vi "Periodic Tasks.vi"(8 "error in":errorcluster) -> ()   [LabVIEW 2015]
doc: "This VI runs in parallel to other tasks. It can contain as many user-defined periodic loops as you need. These can carry out PID or other sorts of timed response."
uses:
  <vilib>/Rock Robotics/WPI/Solenoid/WPI_SolenoidValue.ctl
  <vilib>/Rock Robotics/WPI/Utilities/WPI_GetSetVariantRefNum.vi
  Robot Global Data.vi
  <vilib>/Rock Robotics/WPI/Solenoid/WPI_SolenoidSetEnum.vi
  <vilib>/Rock Robotics/Network Tables/NT Write Number.vi
  <vilib>/Rock Robotics/Network Tables/NT Write Boolean.vi
  <vilib>/Rock Robotics/WPI/Solenoid/Deprecated/WPI_SolenoidGetBool.vi
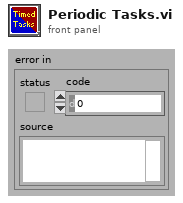
[diagram p1: front panel]
types:
  T1 = typedef "WPI_JoystickDevRef.ctl" = cluster{"Device":T2}
  T2 = typedef "WPI_JoystickDeviceEnum.ctl" = enum16{"USB 0", "USB 1", "USB 2", "USB 3", "USB 4", "USB 5"}
  T3 = typedef "WPI_SolenoidValue.ctl" = enum16{"Off", "On", "Forward", "Reverse"}
  T4 = typedef "WPI_SolenoidDevRef.ctl" = cluster{"DevStatus":errorcluster, "Pneumatics Control Module":u8, "Forward Solenoid Channel":T5, "Reverse Solenoid Channel":T5}
  T5 = typedef "WPI_SolenoidChannel.ctl" = enum8{"Solenoid 0", "Solenoid 1", "Solenoid 2", "Solenoid 3", "Solenoid 4", "Solenoid 5", "Solenoid 6", "Solenoid 7", "Invalid"}
  T6 = typedef "WPI_RobotDriveDevRef.ctl" = cluster{"DevStatus":errorcluster, "Motors[]":T7[], "Square Inputs":bool, "Max Output":dbl}
  T7 = typedef "WPI_MotorControlDeviceRef.ctl" = cluster{"DeviceStatus":errorcluster, "Type":T8, "PWM":cluster{"PWM Channel":T9, "DeadBand":T10}, "CAN":cluster{"Device Number":u8, "Control Mode":T11, "Semaphore":T12, "Max Vout":dbl, "TalonSRX Control Mode":T13}, "Invert":bool}
  T8 = typedef "WPI_MotorControlType.ctl" = enum16{"PWM", "CAN", "CANTalonSRX"}
  T9 = typedef "FPGA_DIOPWMChannel.ctl" = enum8{"PWM 0", "PWM 1", "PWM 2", "PWM 3", "PWM 4", "PWM 5", "PWM 6", "PWM 7", "PWM 8", "PWM 9", "PWM MXP 0", "PWM MXP 1", "PWM MXP 2", "PWM MXP 3", "PWM MXP 4", "PWM MXP 5", "PWM MXP 6", "PWM MXP 7", "PWM MXP 8", "PWM MXP 9", "Invalid"}
  T10 = typedef "WPI_PWMDeadband.ctl" = cluster{"Name":string, "maxPositivePwm":i32, "minPositivePwm":i32, "centerPwm":i32, "maxNegativePwm":i32, "minNegativePwm":i32, "angularRange":u16}
  T11 = typedef "WPI_CANJaguar_ControlMode.ctl" = enum8{"Percent VBus", "Current", "Speed", "Position", "Voltage"}
  T12 = typedef "Semaphore RefNum" = refnum<k1>
  T13 = typedef "WPI_CANTalonSRX_APIControlMode.ctl" = enum8{"Percent VBus", "Speed", "Position", "Slave", "Unchanged / Invalid", "Voltage Compensation", "Current", "Motion Profile"}
  T14 = cluster{"JoystickDevRef":T1, "RobotDriveDevRef":T6}
  T15 = typedef "WPI_CompressorDevRef.ctl" = cluster{"DevStatus":errorcluster, "Pneumatics Control Module":u8}
  T16 = typedef "WPI_DigitalInputDevRef.ctl" = cluster{"DevStatus":errorcluster, "DIO Channel":T17}
  T17 = typedef "FPGA_DIOChannel.ctl" = enum8{"DIO 0", "DIO 1", "DIO 2", "DIO 3", "DIO 4", "DIO 5", "DIO 6", "DIO 7", "DIO 8", "DIO 9", "DIO MXP 0", "DIO MXP 1", "DIO MXP 2", "DIO MXP 3", "DIO MXP 4", "DIO MXP 5", "DIO MXP 6", "DIO MXP 7", "DIO MXP 8", "DIO MXP 9", "DIO MXP 10", "DIO MXP 11", "DIO MXP 12", "DIO MXP 13", "DIO MXP 14", "DIO MXP 15", "Invalid"}
  T18 = typedef "WPI_AnalogChannelDevRef.ctl" = cluster{"DevStatus":errorcluster, "Analog Channel":T19}
  T19 = typedef "FPGA_AIChannel.ctl" = enum8{"AI 0", "AI 1", "AI 2", "AI 3", "AI MXP 0", "AI MXP 1", "AI MXP 2", "AI MXP 3", "Invalid"}
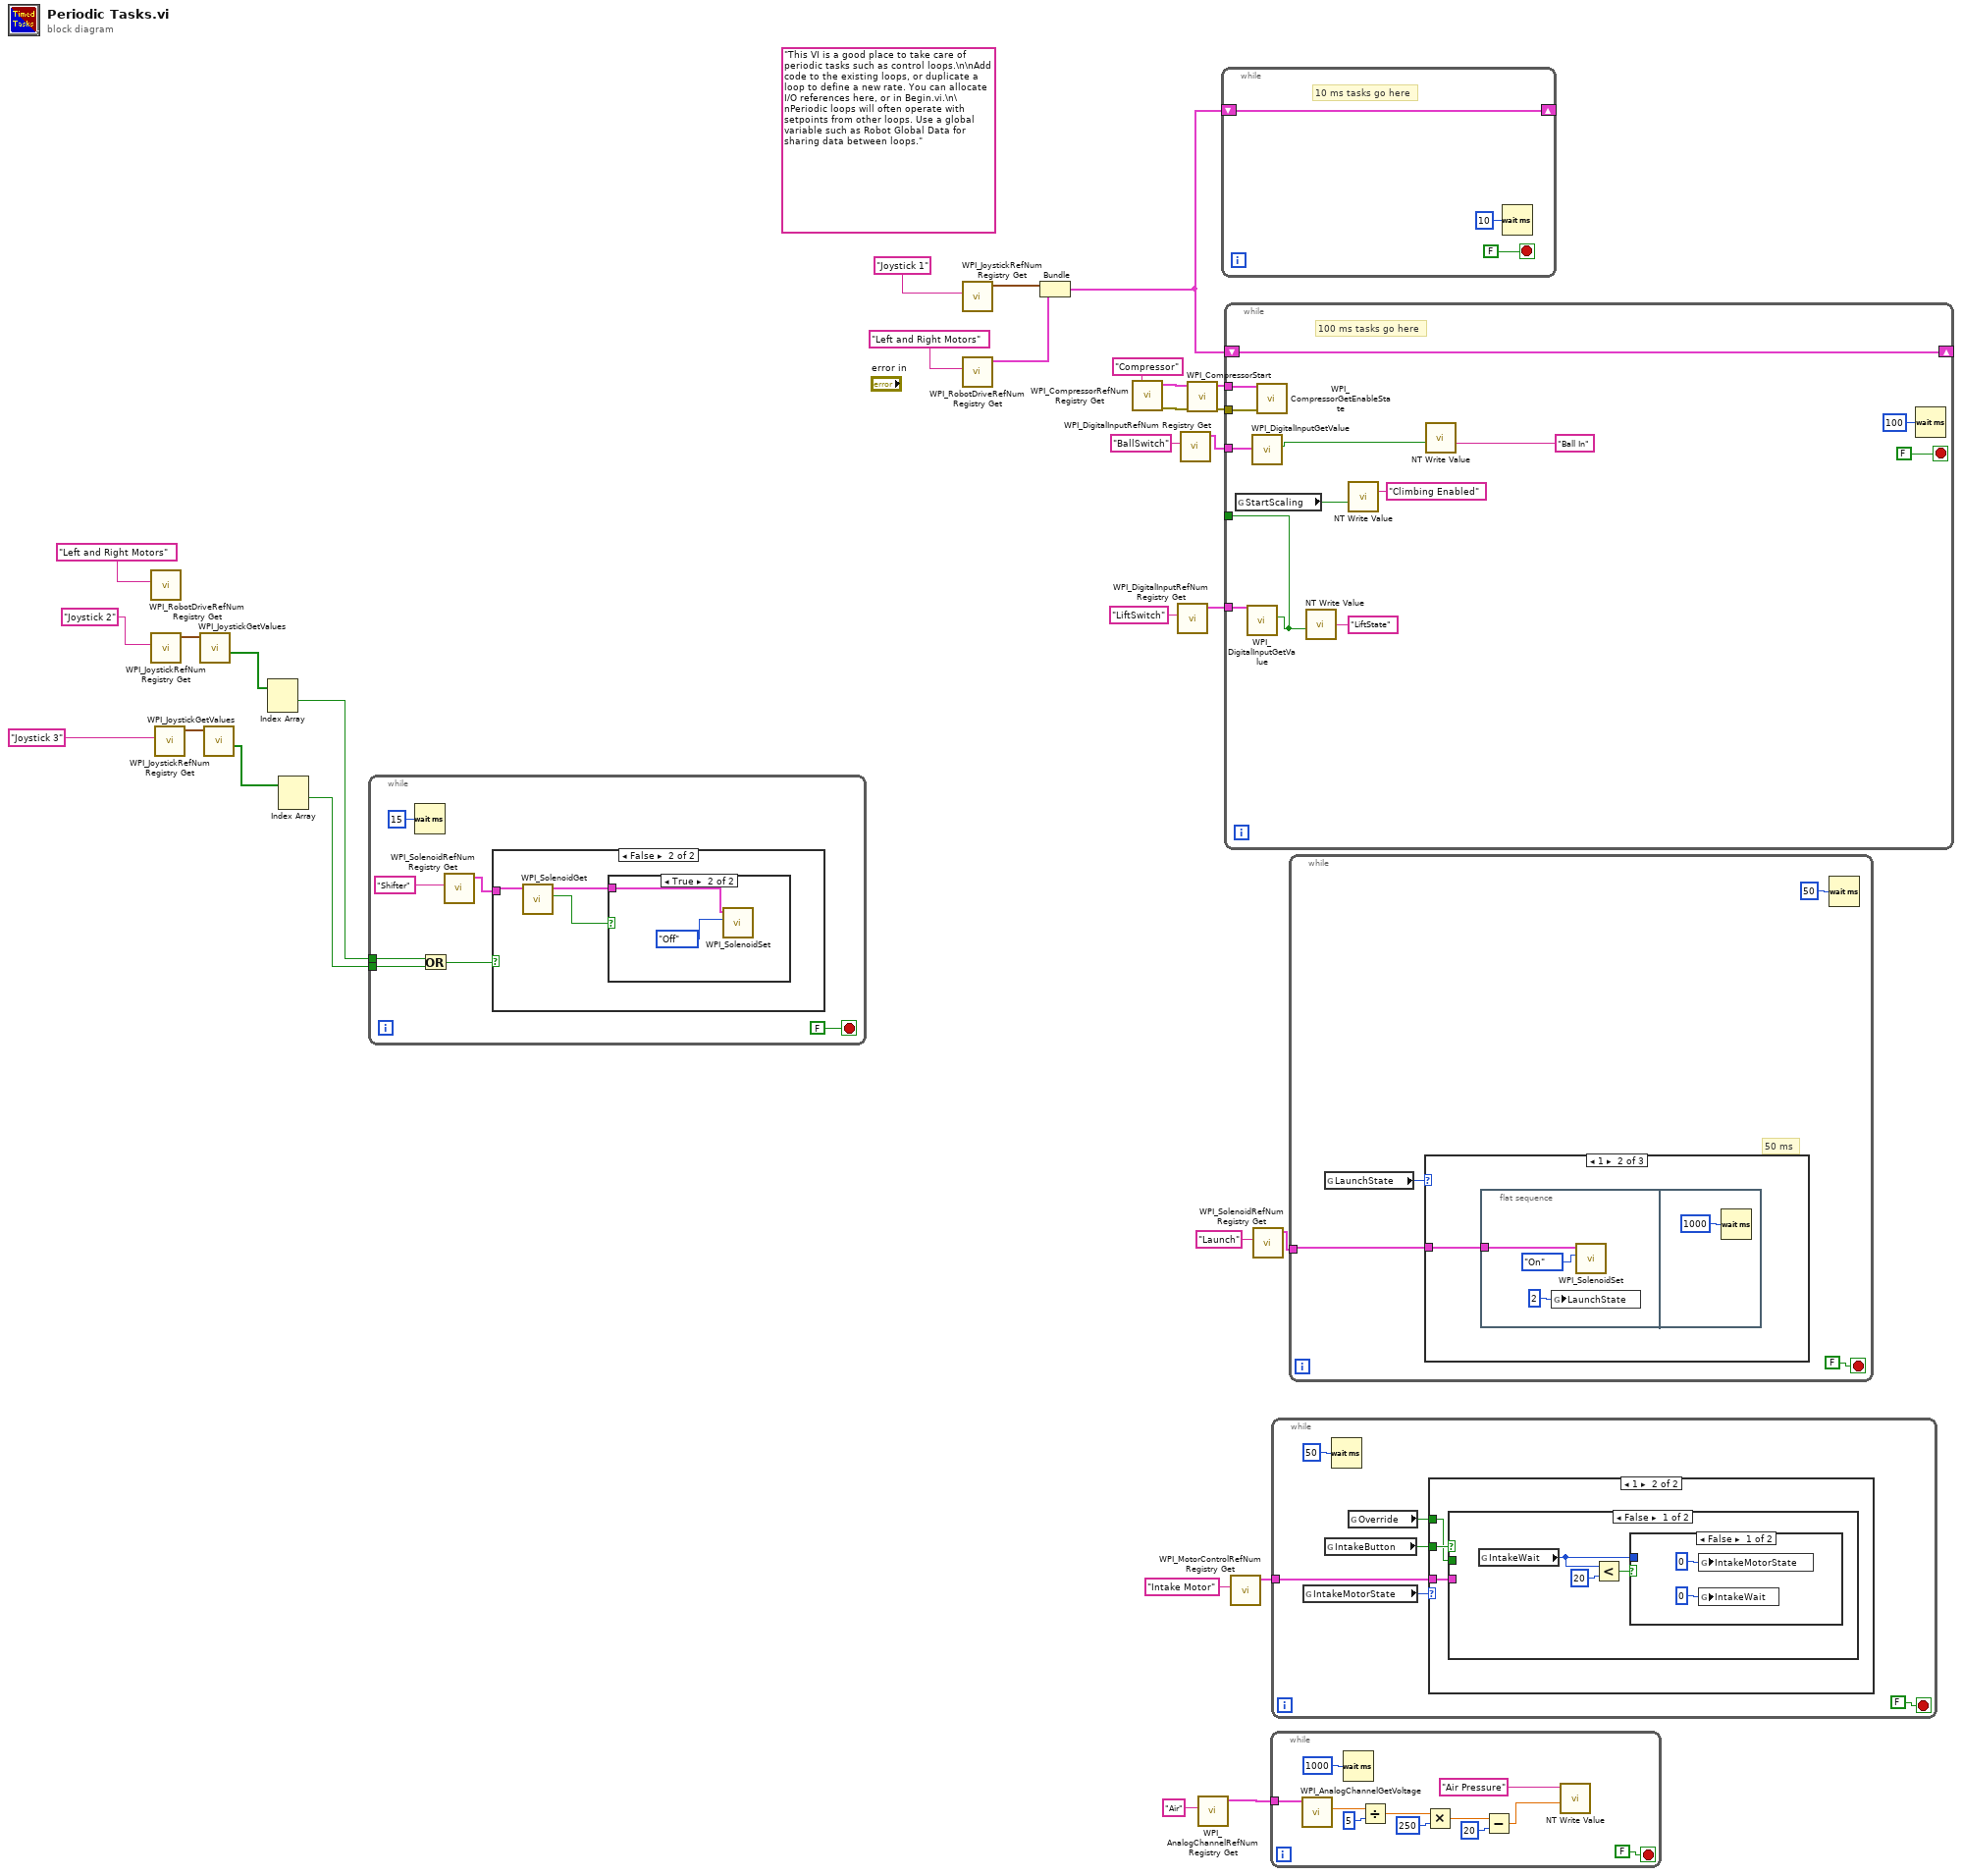
[diagram p0: block diagram]
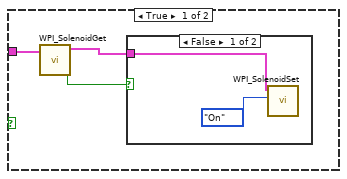
[diagram p2: hidden frame]
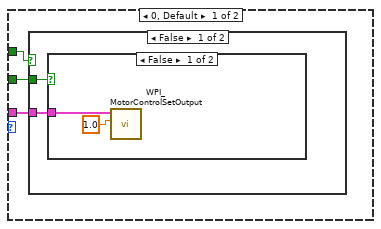
[diagram p5: hidden frame]
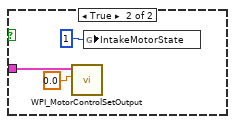
[diagram p6: hidden frame]
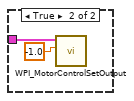
[diagram p7: hidden frame]
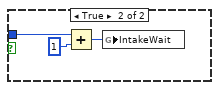
[diagram p8: hidden frame]
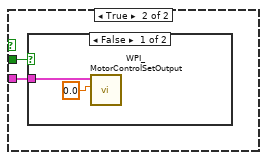
[diagram p9: hidden frame]
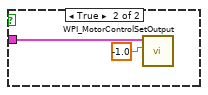
[diagram p10: hidden frame]
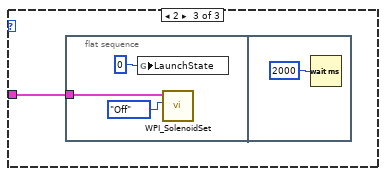
[diagram p12: hidden frame]
diagram:
  (unwired) "This VI is a good place to take care of periodic tasks such as control loops.\n\nAdd code to the existing loops, or duplicate a loop to define a new rate. You can allocate I/O references here, or in Begin.vi.\n\nPeriodic loops will often operate with setpoints from other loops. Use a global variable such as Robot Global Data for sharing data between loops."
  n1 = call <vilib>:"WPI_RobotDriveRefNum Registry Get.vi"("refnum name"="Left and Right Motors") -> ()  [unwired: 1 in, 10 out]
  n2 = call <vilib>:"WPI_JoystickRefNum Registry Get.vi"("refnum name"="Joystick 2") -> ("JoystickDevRef"=w7:T1)  [unwired: 1 in, 9 out]
  n3 = call <vilib>:"WPI_JoystickRefNum Registry Get.vi"("refnum name"="Joystick 3") -> ("JoystickDevRef"=w6:T1)  [unwired: 1 in, 9 out]
  n4 = call <vilib>:"WPI_JoystickGetValues.vi"("JoystickDevRef"=w7) -> ("Buttons"=w4:bool[])  [unwired: 6 in, 4 out]
  n5 = call <vilib>:"WPI_JoystickGetValues.vi"("JoystickDevRef"=w6) -> ("Buttons"=w3:bool[])  [unwired: 6 in, 4 out]
  n6 = Index Array(array=w4) -> (element #1=w2:bool)  [unwired: 2 in, 1 out]
  n7 = Index Array(array=w3) -> (element #1=w1:bool)  [unwired: 2 in, 1 out]
  n8 = while {
    tunnel: w2 -> [w33]
    tunnel: w1 -> [w32]
    stop <- FALSE stop-if-true
    n9 = Wait (ms)(milliseconds to wait=u32 15) -> ()  [unwired: 1 out]
    n10 = Or(x=w33, y=w32) -> (x .or. y?=w34:bool)
    n11 = call <vilib>:"WPI_SolenoidRefNum Registry Get.vi"("refnum name"="Shifter") -> ("SolenoidDevRef"=w36:T4)  [unwired: 9 in, 1 out]
    n12 = case shown="False" w34 {
      tunnel: w36 -> [w37 w42]
      frame True {
        n13 = call-poly <vilib>:"WPI_SolenoidGet.vi"("SolenoidDevRef"=w37) -> ("Value"=w38:bool, "SolenoidDevRef"=w39:T4)  [unwired: 8 in, 1 out]
        n14 = case shown="False" w38 {
          tunnel: w39 -> [w40 _]
          frame False {
            n15 = call-poly <vilib>:"WPI_SolenoidSet.vi"("Value"=WPI_SolenoidValue."On", "SolenoidDevRef"=w40) -> ()  [unwired: 8 in, 2 out]
          }
          frame True {
          }
        }
      }
      frame False {
        n16 = call-poly <vilib>:"WPI_SolenoidGet.vi"("SolenoidDevRef"=w42) -> ("Value"=w43:bool, "SolenoidDevRef"=w44:T4)  [unwired: 8 in, 1 out]
        n17 = case shown="True" w43 {
          tunnel: w44 -> [_ w46]
          frame False {
          }
          frame True {
            n18 = call-poly <vilib>:"WPI_SolenoidSet.vi"("Value"=WPI_SolenoidValue."Off", "SolenoidDevRef"=w46) -> ()  [unwired: 8 in, 2 out]
          }
        }
      }
    }
  }
  n19 = call <vilib>:"WPI_JoystickRefNum Registry Get.vi"("refnum name"="Joystick 1") -> ("JoystickDevRef"=w27:T1)  [unwired: 1 in, 9 out]
  n20 = call <vilib>:"WPI_RobotDriveRefNum Registry Get.vi"("refnum name"="Left and Right Motors") -> ("RobotDriveDevRef"=w26:T6)  [unwired: 1 in, 9 out]
  n21 = Bundle("JoystickDevRef"=w27, "RobotDriveDevRef"=w26) -> (w25:T14)  [unwired: 1 out]
  n22 = call <vilib>:"WPI_CompressorRefNum Registry Get.vi"("refnum name"="Compressor") -> ("error out"=w22:errorcluster, "CompressorDevRef"=w23:T15)  [unwired: 9 in]
  n23 = call <vilib>:"WPI_DigitalInputRefNum Registry Get.vi"("refnum name"="LiftSwitch") -> ("DigitalInputDevRef"=w10:T16)  [unwired: 9 in, 1 out]
  n24 = call <vilib>:"WPI_DigitalInputRefNum Registry Get.vi"("refnum name"="BallSwitch") -> ("DigitalInputDevRef"=w12:T16)  [unwired: 9 in, 1 out]
  n25 = call <vilib>:"WPI_CompressorStart.vi"("error in (no error)"=w22, "CompressorDevRef"=w23) -> ("error out"=w21:errorcluster, "CompressorDevRef"=w24:T15)  [unwired: 8 in]
  n26 = call <vilib>:"WPI_AnalogChannelRefNum Registry Get.vi"("refnum name"="Air") -> ("AIDeviceRef"=w14:T18)  [unwired: 9 in, 1 out]
  n27 = while {
    shift-right: [w47] -> _
    shift-left: w25 -> [w47]
    stop <- FALSE stop-if-true
    # "10 ms tasks go here"
    n28 = Wait (ms)(milliseconds to wait=u32 10) -> ()  [unwired: 1 out]
  }
  n29 = while {
    shift-right: [w60] -> _
    shift-left: w25 -> [w60]
    tunnel: w24 -> [w59]
    tunnel: w21 -> [w58]
    tunnel: w12 -> [w57]
    tunnel: w10 -> [w52]
    tunnel: [w50] -> _
    stop <- FALSE stop-if-true
    # "100 ms tasks go here"
    n30 = global read "Robot Global Data.vi" "StartScaling"() -> (w53:bool)
    n31 = call <vilib>:"WPI_DigitalInputGetValue.vi"("DigitalInputDevRef"=w52) -> ("Value"=w50:bool)  [unwired: 8 in, 2 out]
    n32 = call <vilib>:"WPI_DigitalInputGetValue.vi"("DigitalInputDevRef"=w57) -> ("Value"=w55:bool)  [unwired: 8 in, 2 out]
    n33 = call <vilib>:"WPI_CompressorGetEnableState.vi"("error in (no error)"=w58, "CompressorDevRef"=w59) -> ()  [unwired: 6 in, 4 out]
    n34 = call-poly <vilib>:"NT Write Value.vi"("Boolean"=w50, "Name"="LiftState") -> ()  [unwired: 9 in, 1 out]
    n35 = call-poly <vilib>:"NT Write Value.vi"("Boolean"=w53, "Name"="Climbing Enabled") -> ()  [unwired: 9 in, 1 out]
    n36 = call-poly <vilib>:"NT Write Value.vi"("Boolean"=w55, "Name"="Ball In") -> ()  [unwired: 9 in, 1 out]
    n37 = Wait (ms)(milliseconds to wait=u32 100) -> ()  [unwired: 1 out]
  }
  n38 = call <vilib>:"WPI_MotorControlRefNum Registry Get.vi"("refnum name"="Intake Motor") -> ("MotorControlDevRef"=w16:T7)  [unwired: 9 in, 1 out]
  n39 = call <vilib>:"WPI_SolenoidRefNum Registry Get.vi"("refnum name"="Launch") -> ("SolenoidDevRef"=w18:T4)  [unwired: 9 in, 1 out]
  n40 = while {
    tunnel: w14 -> [w65]
    stop <- FALSE stop-if-true
    n41 = call <vilib>:"WPI_AnalogChannelGetVoltage.vi"("AIDeviceRef"=w65) -> ("Voltage"=w68:dbl)  [unwired: 8 in, 2 out]
    n42 = Wait (ms)(milliseconds to wait=u32 1000) -> ()  [unwired: 1 out]
    n43 = Divide(x=w68, y=5) -> (x/y=w69:dbl)
    n44 = Multiply(x=w69, y=250) -> (x*y=w71:dbl)
    n45 = Subtract(x=w71, y=20) -> (x-y=w73:dbl)
    n46 = call-poly <vilib>:"NT Write Value.vi"("Numeric"=w73, "Name"="Air Pressure") -> ()  [unwired: 9 in, 1 out]
  }
  n47 = while {
    tunnel: w16 -> [w79]
    stop <- FALSE stop-if-true
    n48 = global read "Robot Global Data.vi" "IntakeMotorState"() -> (w75:u8)
    n49 = global read "Robot Global Data.vi" "IntakeButton"() -> (w74:bool)
    n50 = Wait (ms)(milliseconds to wait=u32 50) -> ()  [unwired: 1 out]
    n51 = global read "Robot Global Data.vi" "Override"() -> (w78:bool)
    n52 = case shown="1" w75 {
      tunnel: w79 -> [w82 w94]
      tunnel: w74 -> [w81 w93]
      tunnel: w78 -> [w80 w92]
      frame 0, Default {
        n53 = case shown="False" w80 {
          tunnel: w82 -> [w84 w90]
          tunnel: w81 -> [w83 _]
          frame False {
            n54 = case shown="False" w83 {
              tunnel: w84 -> [w85 w87]
              frame False {
                n55 = call <vilib>:"WPI_MotorControlSetOutput.vi"("Output"=1.0, "MotorControlDevRef"=w85) -> ()  [unwired: 7 in, 3 out]
              }
              frame True {
                n56 = call <vilib>:"WPI_MotorControlSetOutput.vi"("Output"=0.0, "MotorControlDevRef"=w87) -> ()  [unwired: 7 in, 3 out]
                n57 = global write "Robot Global Data.vi" "IntakeMotorState"(u8 1 ("LaunchState")) -> ()
              }
            }
          }
          frame True {
            n58 = call <vilib>:"WPI_MotorControlSetOutput.vi"("Output"=-1.0, "MotorControlDevRef"=w90) -> ()  [unwired: 7 in, 3 out]
          }
        }
      }
      frame 1 {
        n59 = case shown="False" w93 {
          tunnel: w94 -> [_ w104]
          tunnel: w92 -> [_ w103]
          frame False {
            n60 = global read "Robot Global Data.vi" "IntakeWait"() -> (w95:u8)
            n61 = Less?(x=w95, y=u8 20) -> (x < y?=w96:bool)
            n62 = case shown="False" w96 {
              tunnel: w95 -> [_ w102]
              frame False {
                n63 = global write "Robot Global Data.vi" "IntakeMotorState"(u8 0 ("IntakeMotorState")) -> ()
                n64 = global write "Robot Global Data.vi" "IntakeWait"(u8 0 ("IntakeWait")) -> ()
              }
              frame True {
                n65 = Add(x=w102, y=u8 1) -> (x+y=w100:u8)
                n66 = global write "Robot Global Data.vi" "IntakeWait"(w100) -> ()
              }
            }
          }
          frame True {
            n67 = case shown="False" w103 {
              tunnel: w104 -> [w105 w107]
              frame False {
                n68 = call <vilib>:"WPI_MotorControlSetOutput.vi"("Output"=0.0, "MotorControlDevRef"=w105) -> ()  [unwired: 7 in, 3 out]
              }
              frame True {
                n69 = call <vilib>:"WPI_MotorControlSetOutput.vi"("Output"=-1.0, "MotorControlDevRef"=w107) -> ()  [unwired: 7 in, 3 out]
              }
            }
          }
        }
      }
    }
  }
  n70 = while {
    tunnel: w18 -> [w111]
    stop <- FALSE stop-if-true
    # "50 ms"
    n71 = global read "Robot Global Data.vi" "LaunchState"() -> (w112:u8)
    n72 = case shown="1" w112 {
      tunnel: w111 -> [_ w113 w118]
      frame 0, Default {
      }
      frame 1 {
        n73 = flat-sequence {
          tunnel: w113 -> [w114]
          frame #0 {
            n74 = global write "Robot Global Data.vi" "LaunchState"(u8 2 ("LaunchState")) -> ()
            n75 = call-poly <vilib>:"WPI_SolenoidSet.vi"("Value"=WPI_SolenoidValue."On", "SolenoidDevRef"=w114) -> ()  [unwired: 8 in, 2 out]
          }
          frame #1 {
            n76 = Wait (ms)(milliseconds to wait=u32 1000) -> ()  [unwired: 1 out]
          }
        }
      }
      frame 2 {
        n77 = flat-sequence {
          tunnel: w118 -> [w119]
          frame #0 {
            n78 = global write "Robot Global Data.vi" "LaunchState"(u8 0 ("LaunchState")) -> ()
            n79 = call-poly <vilib>:"WPI_SolenoidSet.vi"("Value"=WPI_SolenoidValue."Off", "SolenoidDevRef"=w119) -> ()  [unwired: 8 in, 2 out]
          }
          frame #1 {
            n80 = Wait (ms)(milliseconds to wait=u32 2000) -> ()  [unwired: 1 out]
          }
        }
      }
    }
    n81 = Wait (ms)(milliseconds to wait=u32 50) -> ()  [unwired: 1 out]
  }
